vi "LVClass_Camera stop acquisition.vi"(0 "Camera in":refnum<class "Camera.lvclass">, 11 "error in (no error)":errorcluster) -> (4 "Camera out":refnum<class "Camera.lvclass">, 15 "error out":errorcluster)   [LabVIEW 2020, in "Camera.lvclass"]
doc: "Stop acquisition.\n\n<B>CameraIn</B> : Camera object.\n<B>CameraOut</B> : Camera object."
uses:
  Camera.lvclass
  CameraAcquisitionState.ctl
  Camera.lvclass/Camera.ctl
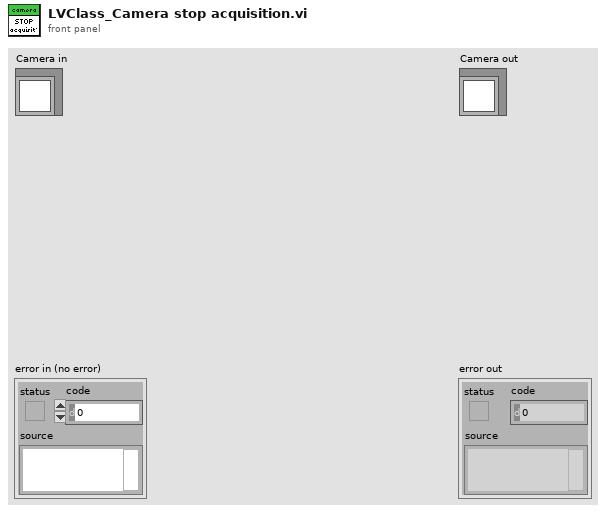
[diagram p1: front panel]
types:
  T1 = typedef "CameraAcquisitionState.ctl" = enum16{"Stop", "Live"}
  T2 = typedef "ClassID.ctl" = i64
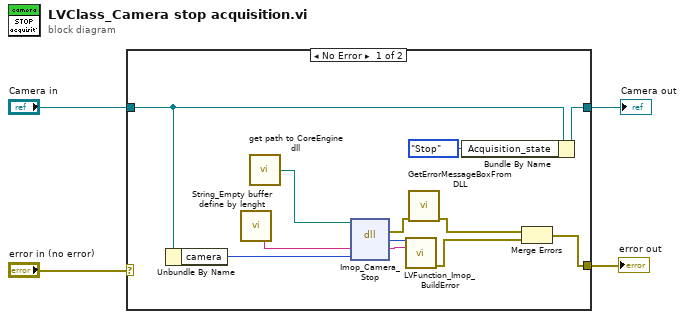
[diagram p0: block diagram]
diagram:
  n1 = case shown="No Error" "error in (no error)" {
    selector: "error in (no error)" -> [_ w18]
    tunnel: [w8 w18] -> w3
    tunnel: [w6 w17] -> w1
    tunnel: "Camera in" -> [w7 w17]
    frame No Error {
      n2 = Unbundle By Name(w7) -> ("camera"=w15:T2)
      n3 = call "String_Empty buffer define by lenght.vi"() -> ("Empty buffer"=w16:string)  [unwired: 1 in]
      n4 = call "get path to CoreEngine dll.vi"() -> ("path to wavekit library"=w12:path)  [unwired: 14 in, 1 out]
      n5 = dll-call lib="D:/2_trunk/Soft_haso/ImOpCoreEngine4_LV2011/DLLs/ImopEngine4_vc100.dll" fn="Imop_Camera_Stop"(path in=w12, "message"=w16, "objet"=w15) -> (error out=w11:errorcluster, "return type"=w13:i32, "message"=w14:string)  [unwired: 3 in, 1 out]
      n6 = call "LVFunction_Imop_BuildError.vi"("code"=w13, "String to Prepend to source (\"\")"=w14) -> ("error out"=w9:errorcluster)  [unwired: 13 in]
      n7 = call "GetErrorMessageBoxFromDLL.vi"("error IN"=w11) -> ("error OUT"=w10:errorcluster)  [unwired: 10 in]
      n8 = Bundle By Name(cluster=w7, "Acquisition_state"=CameraAcquisitionState."Stop") -> (w6:refnum<class "Camera.lvclass">)
      n9 = Merge Errors(w10, w9) -> (w8:errorcluster)
    }
    frame Error {
    }
  }
  "error out" <- w3
  "Camera out" <- w1
